vi "功能计算_何.vi"(8 "截取%":i32, 9 "索引":i32=17, 10 "扭矩数组":dbl[](array[numeric])) -> (0 "扭差":dbl format="%#.2f", 1 "平均扭矩":dbl format="%#.2f", 2 "最小扭矩":dbl, 3 "峰值扭矩":dbl format="%#.2f")   [LabVIEW 2013]
panel:
  out "第一个子数组":dbl[](array[numeric])
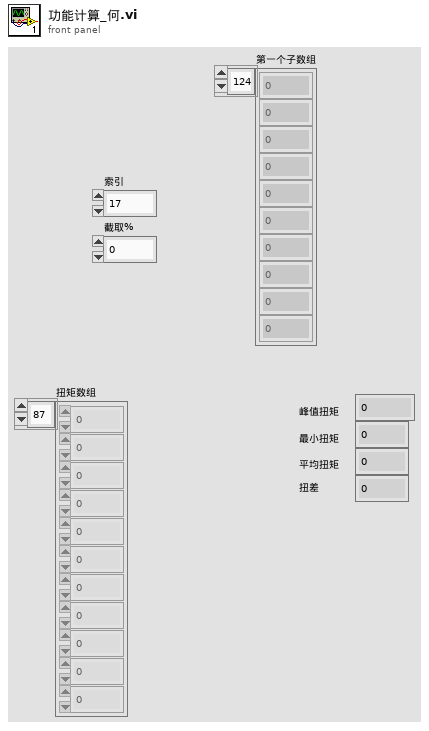
[diagram p1: front panel]
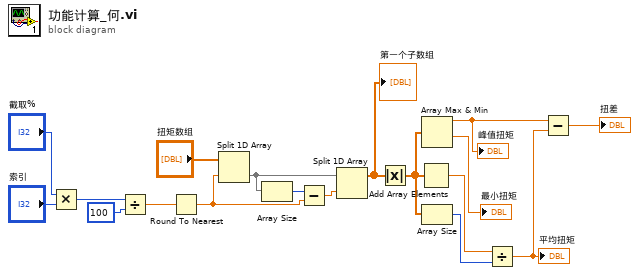
[diagram p0: block diagram]
diagram:
  n1 = Multiply(x="截取%", y="索引") -> (x*y=w4:i32)
  n2 = Divide(x=w4, y=100) -> (x/y=w2:dbl)
  n3 = Round To Nearest(number=w2) -> (nearest integer value=w3:dbl)
  n4 = Split 1D Array(array="扭矩数组", index=w3) -> (second subarray=w10:dbl[])  [unwired: 1 out]
  n5 = Array Size(array=w10) -> (size(s)=w9:i32)
  n6 = Subtract(x=w9, y=w3) -> (x-y=w8:dbl)
  n7 = Split 1D Array(array=w10, index=w8) -> (first subarray=w14:dbl[])  [unwired: 1 out]
  "第一个子数组" <- w14
  n8 = Absolute Value(x=w14) -> (abs(x)=w16:dbl[])
  n9 = Add Array Elements(numeric array=w16) -> (sum=w17:dbl)
  n10 = Array Max & Min(array=w16) -> (max value=w13:dbl, min value=→"最小扭矩":dbl)  [unwired: 2 out]
  "峰值扭矩" <- w13
  n11 = Array Size(array=w16) -> (size(s)=w15:i32)
  n12 = Divide(x=w17, y=w15) -> (x/y=w12:dbl)
  "平均扭矩" <- w12
  n13 = Subtract(x=w13, y=w12) -> (x-y=→"扭差":dbl)
